vi "runscenario process nonPDF.vi"(5 "Raw Text Content (\"\")":string) -> (2 "Processed Template Content":string)   [LabVIEW 2011]
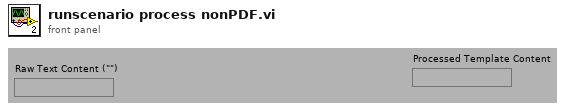
[diagram p1: front panel]
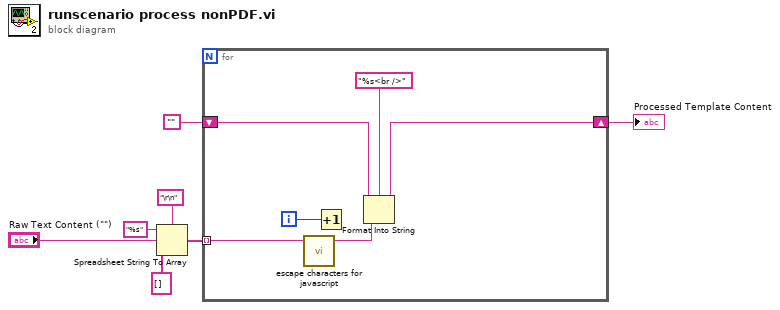
[diagram p0: block diagram]
diagram:
  n1 = Spreadsheet String To Array(delimiter (Tab)="\r\n" ("search string"), format string="%s", spreadsheet string="Raw Text Content (\"\")", array type (2D Dbl)=string[] []) -> (array=w4:string[])
  n2 = for {
    tunnel: w4 -> [w9] mode=indexing
    shift-right: [w10] -> w2
    shift-left: "" -> [w11]
    i -> [w12]
    n3 = call "escape characters for javascript.vi"("String (\"\")"=w9) -> ("escaped String"=w8:string)  [unwired: 4 out]
    n4 = Increment(x=w12) -> ()  [unwired: 1 out]
    n5 = Format Into String(format string="%s<br />" ("delimiter (Tab)"), initial string=w11, w8) -> (resulting string=w10:string)  [unwired: 1 in, 1 out]
  }
  "Processed Template Content" <- w2
